vi "Main.vi"() -> ()   [LabVIEW 2021]
doc: "This vi acts as an user interface to display acquire data and save data when required. User can ineract with the panel to choose file (CSV or TDMS) and data display type(chart or graph). It also allow user to select channel index and define channel name, scale and offset. It then can let user choose a moment to start recording either on defined time length or user choice."
uses:
  Control/Data Display Choice Enum.ctl
  Control/File Choice Enum.ctl
  Control/User Interface Reference Cluster.ctl
  Control/Data Display Manager Enum.ctl
  Control/Volt Chl.ctl
  Control/File Manager Enum.ctl
  Control/Command and Data Cluster.ctl
  Control/DAQ Manager Enum.ctl
  <extravilib>/ChannelInstances/Stream-a[.](wfm(dbl))/Read With Abort.vi
  <extravilib>/ChannelInstances/Stream-a[.](wfm(dbl))/Write With Abort.vi
  <extravilib>/ChannelInstances/Stream-a[.](wfm(dbl))/EndpointRead.vi
  <extravilib>/ChannelInstances/Stream-a[.](wfm(dbl))/Endpoint.vi
  <extravilib>/ChannelInstances/Stream-a[.](wfm(dbl))/Instantiate.vi
  <extravilib>/ChannelInstances/Event Messenger-t'Command and Data Cluster.ctl'/Instantiate.vi
  <extravilib>/ChannelInstances/Event Messenger-t'Command and Data Cluster.ctl'/))Channel.vi
  <extravilib>/ChannelInstances/Stream-a[.](wfm(dbl))/)Channel.vi
  <resource>/ChannelSupport/_ChannelSupport/WaitIfNeeded.vi
  <extravilib>/ChannelInstances/Event Messenger-t'Command and Data Cluster.ctl'.lvlib
  <extravilib>/ChannelInstances/Stream-a[.](wfm(dbl)).lvlib
panel:
  out "Error":errorcluster
  out "Overall Raw \nVoltage Mean":dbl[](array[numeric])
  out "Raw Voltage Mean \nper Second":dbl[](array[numeric])
  out "Recording":bool
  in  "File Choice":T1=enum."CSV File"
  in  "DD Choice":T2 caption="Data Display Choice"
  out "File Path":path
  in  "Choice Ok":bool
  in  "File Name":string
  in  "Exit":bool
  in  "Use Re Time":bool caption="Use Record Time"
  in  "Re Time":dbl=10.0 caption="Record Time (s)"
  in  "Device Name":tag
  in  "Sample Rate":i32=100 caption="Sample Rate (S/s)"
  in  "Init Button":bool
  in  "Record":bool
  in  "Start":bool
  in  "Stop":bool
  out "element":waveform(dbl)[](array[waveform])
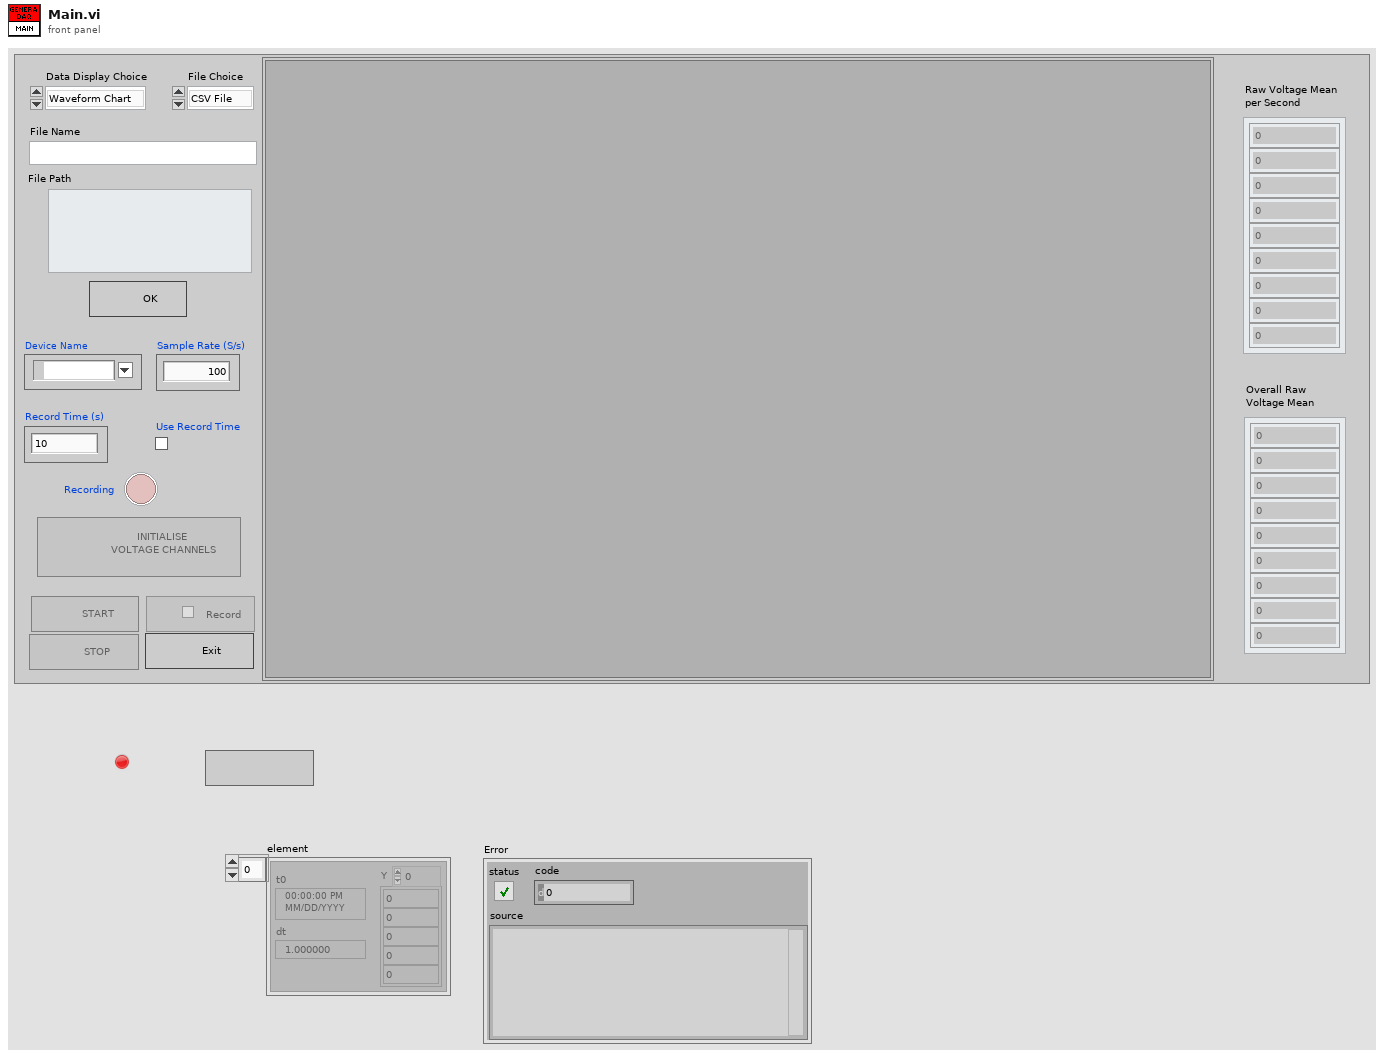
[diagram p1: front panel]
types:
  T1 = typedef "File Choice Enum.ctl" = enum16{"TDMS File", "CSV File"}
  T2 = typedef "Data Display Choice Enum.ctl" = enum16{"Waveform Chart", "Waveform Graph"}
  T3 = typedef "User Interface Reference Cluster.ctl" = cluster{"Choice Ok":refnum<vi>, "Init Button":refnum<vi>, "Start":refnum<vi>, "Record":refnum<vi>, "Stop":refnum<vi>, "Exit":refnum<vi>, "File Choice":refnum<vi>, "DD Choice":refnum<vi>}
  T4 = typedef "Command and Data Cluster.ctl" = cluster{"Command":string, "Data":variant}
  T5 = typedef "Event Messenger-t'Command and Data Cluster.ctl'.lvlib/))Channel.ctl" = refnum<queue>
  T6 = typedef "DAQ Manager Enum.ctl" = enum16{"Config", "Start", "Read", "Stop"}
  T7 = typedef "Volt Chl.ctl" = cluster{"Index":i32[], "Chl Name":string[], "Scale":dbl[], "Offset":dbl[], "Sample Rate":i32, "Device Name":tag, "Channel":tag}
  T8 = typedef "Stream-a[.](wfm(dbl)).lvlib/)Channel.ctl" = refnum<queue>
  T9 = typedef "File Manager Enum.ctl" = enum16{"Create File", "Config Data", "Volt Data", "Set Time", "Close File"}
  T10 = typedef "Data Display Manager Enum.ctl" = enum16{"Display Choice", "Config Data", "Volt Data"}
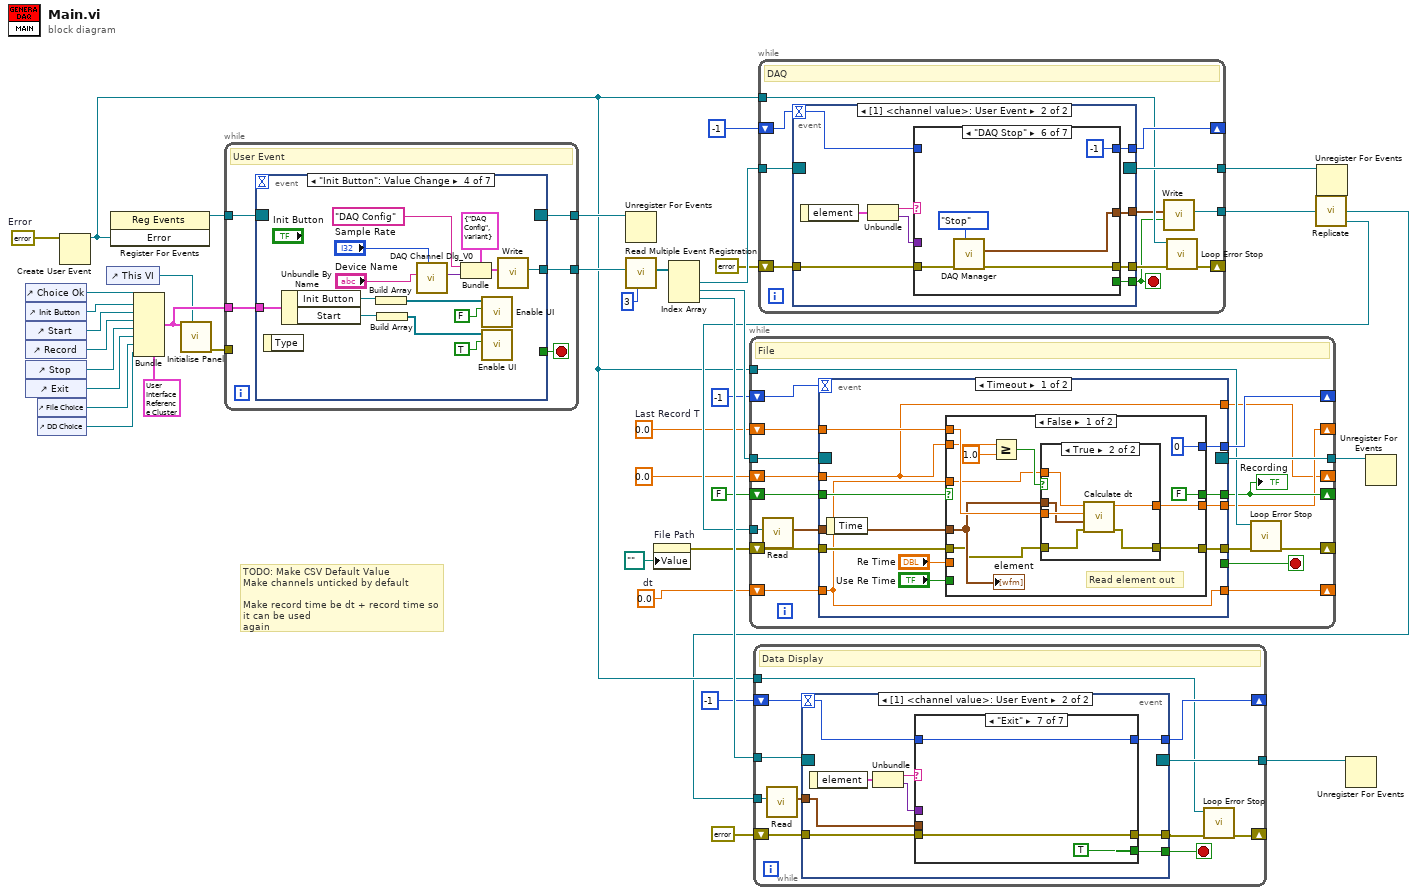
[diagram p0: block diagram]
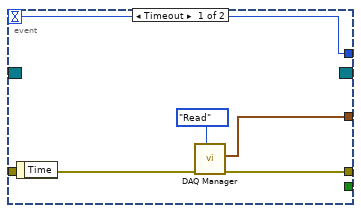
[diagram p2: hidden frame]
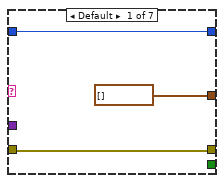
[diagram p3: hidden frame]
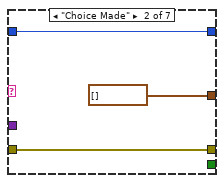
[diagram p4: hidden frame]
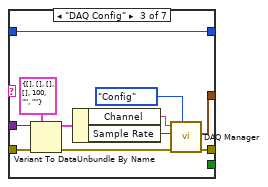
[diagram p5: hidden frame]
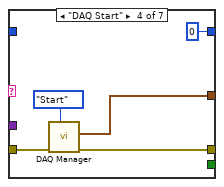
[diagram p6: hidden frame]
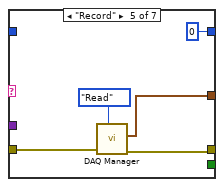
[diagram p7: hidden frame]
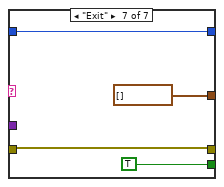
[diagram p8: hidden frame]
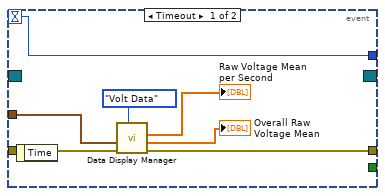
[diagram p9: hidden frame]
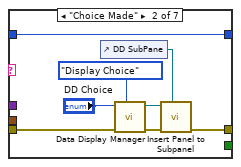
[diagram p11: hidden frame]
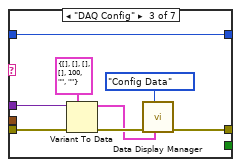
[diagram p12: hidden frame]
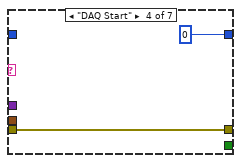
[diagram p13: hidden frame]
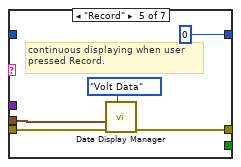
[diagram p14: hidden frame]
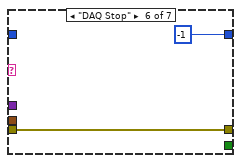
[diagram p15: hidden frame]
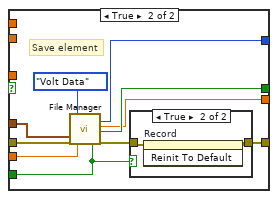
[diagram p17: hidden frame]
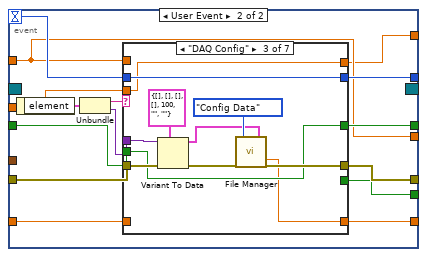
[diagram p19: hidden frame]
diagram:
  w2 = 0.0  # dt
  w3 = 0.0  # Last Record T
  w7 = errorcluster {"status"=FALSE, "code"=0, "source"=""}  # Error
  # "TODO: Make CSV Default Value\nMake channels unticked by default\n\nMake record time be dt + record time so it can be used \nagain"
  n1 = control-ref of="Choice Ok"() -> (w25:refnum<vi>)
  n2 = control-ref of="Init Button"() -> (w24:refnum<vi>)
  n3 = control-ref of="Start"() -> (w23:refnum<vi>)
  n4 = control-ref of="Record"() -> (w22:refnum<vi>)
  n5 = control-ref of="Stop"() -> (w21:refnum<vi>)
  n6 = control-ref of="Exit"() -> (w20:refnum<vi>)
  n7 = control-ref of="File Choice"() -> (w19:refnum<vi>)
  n8 = control-ref of="DD Choice"() -> (w18:refnum<vi>)
  n9 = Create User Event(user event datatype=w7) -> (user event=w10:refnum<user-event>)  [unwired: 1 in, 1 out]
  n10 = control-ref of="This VI"() -> (w8:refnum<vi>)
  n11 = register-events(w10) -> (reference out=w12:refnum<event-registration>)  [unwired: 2 in, 1 out]
  n12 = Bundle(cluster=T3 {"Choice Ok"=refnum, "Init Button"=refnum, "Start"=refnum, "Record"=refnum, "Stop"=refnum, "Exit"=refnum, "File Choice"=refnum, "DD Choice"=refnum} ("output cluster"), "Choice Ok"=w25, "Init Button"=w24, "Start"=w23, "Record"=w22, "Stop"=w21, "Exit"=w20, "File Choice"=w19, "DD Choice"=w18) -> (w15:T3)
  n13 = call "Initialise Panel.vi"("This VI"=w8, "UI Ref"=w15) -> ("error out"=w16:errorcluster)  [unwired: 9 in]
  n14 = while {
    tunnel: [w43] -> w33
    tunnel: w16 -> [_]
    tunnel: w15 -> [w42]
    tunnel: w12 -> [w41]
    tunnel: [w40] -> w11
    stop <- w44 stop-if-true
    # "User Event"
    n15 = event shown="[3] \"Init Button\": Value Change" {
      selector: w41 -> [_ _ _ _ _ _ _]
      dyn-events: [_ _ _ _ _ _ _] -> w40
      timeout: _ -> [_ _ _ _ _ _ _]
      tunnel: [TRUE TRUE _ _ _ _ _] -> w44
      tunnel: [w45 w53 w65 w78 w91 w96 w108] -> w43
      tunnel: w42 -> [_ _ w64 w73 w83 _ w107]
      event "Exit": Value Change {
        n16 = event-data() -> ()  [unwired: 1 in, 1 out]
        n17 = call <extravilib>:"Write.vi"("element"=T4 {"Command"="Exit", "Data"=variant} ("Cluster")) -> ("channel"=w45:T5)  [unwired: 9 in, 1 out]
      }
      event User Event {
        w52 = errorcluster {"status"=FALSE, "code"=0, "source"=""}  # Error
        n18 = event-data() -> ("status"=w51:bool, "code"=w50:i32, "source"=w49:string)  [unwired: 1 in]
        n19 = Bundle(cluster=w52, "status"=w51, "code"=w50, "source"=w49) -> (→"Error":errorcluster)
        n20 = call <extravilib>:"Write.vi"("element"=T4 {"Command"="Exit", "Data"=variant} ("Cluster")) -> ("channel"=w53:T5)  [unwired: 9 in, 1 out]
      }
      event "Choice Ok": Value Change {
        n21 = event-data() -> ()  [unwired: 1 in, 1 out]
        n22 = Unbundle By Name(w64) -> ("File Choice"=w57:refnum<vi>, "DD Choice"=w56:refnum<vi>, "Choice Ok"=w63:refnum<vi>, "Init Button"=w62:refnum<vi>)
        n23 = Build Array(w57, w56, w63) -> (w60:refnum<vi>[])
        n24 = Build Array(w62) -> (w58:refnum<vi>[])
        n25 = call <extravilib>:"Write.vi"("element"=T4 {"Command"="Choice Made", "Data"=variant} ("Cluster")) -> ("channel"=w65:T5)  [unwired: 9 in, 1 out]
        n26 = call "Enable UI.vi"("Enable?"=FALSE, "output cluster"=w60) -> ()  [unwired: 9 in, 1 out]
        n27 = call "Enable UI.vi"("Enable?"=TRUE, "output cluster"=w58) -> ()  [unwired: 9 in, 1 out]
      }
      event "Init Button": Value Change {
        n28 = event-data() -> ()  [unwired: 1 in, 1 out]
        n29 = Unbundle By Name(w73) -> ("Init Button"=w68:refnum<vi>, "Start"=w67:refnum<vi>)
        n30 = Build Array(w68) -> (w72:refnum<vi>[])
        n31 = Build Array(w67) -> (w71:refnum<vi>[])
        n32 = call "DAQ Channel Dlg_V0.vi"("DAQ Sample Rate (S/s)"="Sample Rate", "Device Name"="Device Name") -> ("Chl Infor"=w74:variant)  [unwired: 9 in]
        n33 = Bundle(cluster=T4 {"Command"="DAQ Config", "Data"=variant} ("Cluster"), "Command"="DAQ Config" ("element"), "Data"=w74) -> (w76:T4)
        n34 = call "Enable UI.vi"("Enable?"=FALSE, "output cluster"=w72) -> ()  [unwired: 9 in, 1 out]
        n35 = call "Enable UI.vi"("Enable?"=TRUE, "output cluster"=w71) -> ()  [unwired: 9 in, 1 out]
        n36 = call <extravilib>:"Write.vi"("element"=w76) -> ("channel"=w78:T5)  [unwired: 9 in, 1 out]
      }
      event "Start": Value Change {
        n37 = event-data() -> ()  [unwired: 1 in, 1 out]
        n38 = Unbundle By Name(w83) -> ("Exit"=w81:refnum<vi>, "Start"=w85:refnum<vi>, "Record"=w84:refnum<vi>, "Stop"=w82:refnum<vi>)
        n39 = Build Array(w81, w85) -> (w89:refnum<vi>[])
        n40 = Build Array(w84, w82) -> (w88:refnum<vi>[])
        n41 = call "Enable UI.vi"("Enable?"=FALSE, "output cluster"=w89) -> ()  [unwired: 9 in, 1 out]
        n42 = call "Enable UI.vi"("Enable?"=TRUE, "output cluster"=w88) -> ()  [unwired: 9 in, 1 out]
        n43 = call <extravilib>:"Write.vi"("element"=T4 {"Command"="DAQ Start", "Data"=variant} ("Cluster")) -> ("channel"=w91:T5)  [unwired: 9 in, 1 out]
      }
      event "Record": Value Change {
        n44 = event-data() -> ()  [unwired: 1 in, 1 out]
        n45 = To Variant(anything="Record") -> (Variant=w93:variant)
        n46 = Bundle(cluster=T4 {"Command"="Record", "Data"=variant} ("Cluster"), "Data"=w93) -> (w92:T4)  [unwired: 1 in]
        n47 = call <extravilib>:"Write.vi"("element"=w92) -> ("channel"=w96:T5)  [unwired: 9 in, 1 out]
      }
      event "Stop": Value Change {
        n48 = event-data() -> ()  [unwired: 1 in, 1 out]
        n49 = Unbundle By Name(w107) -> ("Choice Ok"=w103:refnum<vi>, "File Choice"=w104:refnum<vi>, "DD Choice"=w105:refnum<vi>, "Exit"=w101:refnum<vi>, "Record"=w100:refnum<vi>, "Stop"=w97:refnum<vi>)
        n50 = Build Array(w103, w104, w105, w101) -> (w102:refnum<vi>[])
        n51 = Build Array(w100, w97) -> (w98:refnum<vi>[])
        n52 = call "Enable UI.vi"("Enable?"=TRUE, "output cluster"=w102) -> ()  [unwired: 9 in, 1 out]
        n53 = call "Enable UI.vi"("Enable?"=FALSE, "output cluster"=w98) -> ()  [unwired: 9 in, 1 out]
        n54 = call <extravilib>:"Write.vi"("element"=T4 {"Command"="DAQ Stop", "Data"=variant} ("Cluster")) -> ("channel"=w108:T5)  [unwired: 9 in, 1 out]
      }
    }
  }
  n55 = Unregister For Events(event registration refnum=w11) -> ()  [unwired: 1 in, 1 out]
  n56 = call <extravilib>:"Read Multiple Event Registration.vi"("number of event structures"=u16 3, "channel"=w33) -> ("event registration refnums"=w31:refnum<event-registration>[])  [unwired: 9 in]
  n57 = property on="File Path" class="Path"("Value"=path "" ("File Path")) -> (error out=w13:errorcluster)  [unwired: 2 in, 1 out]
  n58 = Index Array(array=w31) -> (element #1=w37:refnum<event-registration>, element #2=w38:refnum<event-registration>, element #3=w36:refnum<event-registration>)  [unwired: 3 in]
  n59 = while {
    tunnel: w37 -> [w120]
    tunnel: [w119] -> w34
    shift-right: [w117] -> _
    shift-left: -1 -> [w118]
    tunnel: [w112] -> w28
    shift-right: [w114] -> _
    shift-left: errorcluster {"status"=FALSE, "code"=0, "source"=""} ("error constant") -> [w116]
    tunnel: w10 -> [w115]
    stop <- w110 stop-if-true
    # "DAQ"
    n60 = event shown="[1] <channel value>: User Event" {
      selector: w120 -> [_ _]
      dyn-events: [_ _] -> w119
      timeout: w118 -> [w125 w129]
      tunnel: [w124 w134] -> w113
      tunnel: [_ w133] -> w110
      tunnel: [w125 w128] -> w117
      tunnel: w116 -> [w122 w127]
      tunnel: [w121 w126] -> w111
      event Timeout {
        n61 = event-data() -> ()  [unwired: 1 in, 1 out]
        n62 = call "DAQ Manager.vi"("Enum"=DAQ_Manager_Enum."Read", "error in"=w122) -> ("error out"=w124:errorcluster, "data"=w121:waveform(dbl)[])  [unwired: 8 in]
      }
      event User Event {
        n63 = event-data() -> ("element"=w132:T4)  [unwired: 1 in]
        n64 = Unbundle(w132) -> ("Command"=w131:string, "Data"=w130:variant)
        n65 = case shown="\"DAQ Stop\"" w131 {
          tunnel: [w136 w139 w144 w155 w157 w164 w168] -> w134
          tunnel: [_ _ _ _ _ _ TRUE] -> w133
          tunnel: w130 -> [_ _ w151 _ _ _ _]
          tunnel: w129 -> [w137 w140 w143 _ _ _ w170]
          tunnel: [w137 w140 w143 0 0 -1 w170] -> w128
          tunnel: w127 -> [w136 w139 w142 w153 w158 w163 w168]
          tunnel: [waveform(dbl)[] [] ("element") waveform(dbl)[] [] ("element") w141 w152 w159 w162 waveform(dbl)[] [] ("element")] -> w126
          frame Default {
          }
          frame "Choice Made" {
          }
          frame "DAQ Config" {
            n66 = Variant To Data(error in=w142, type=T7 {"Index"=[], "Chl Name"=[], "Scale"=[], "Offset"=[], "Sample Rate"=100, "Device Name"="", "Channel"=""} ("Volt Channel"), Variant=w151) -> (data=w149:T7, error out=w146:errorcluster)
            n67 = Unbundle By Name(w149) -> ("Channel"=w148:tag, "Sample Rate"=w147:i32)
            n68 = call "DAQ Manager.vi"("Enum"=DAQ_Manager_Enum."Config", "error in"=w146, "Sample Rate"=w147, "Chl"=w148) -> ("error out"=w144:errorcluster, "data"=w141:waveform(dbl)[])  [unwired: 6 in]
          }
          frame "DAQ Start" {
            n69 = call "DAQ Manager.vi"("Enum"=DAQ_Manager_Enum."Start", "error in"=w153) -> ("error out"=w155:errorcluster, "data"=w152:waveform(dbl)[])  [unwired: 8 in]
          }
          frame "Record" {
            n70 = call "DAQ Manager.vi"("Enum"=DAQ_Manager_Enum."Read", "error in"=w158) -> ("error out"=w157:errorcluster, "data"=w159:waveform(dbl)[])  [unwired: 8 in]
          }
          frame "DAQ Stop" {
            n71 = call "DAQ Manager.vi"("Enum"=DAQ_Manager_Enum."Stop", "error in"=w163) -> ("error out"=w164:errorcluster, "data"=w162:waveform(dbl)[])  [unwired: 8 in]
          }
          frame "Exit" {
          }
        }
      }
    }
    n72 = call <extravilib>:"Write.vi"("last element? (F)"=w110, "element"=w111) -> ("channel"=w112:T8)  [unwired: 7 in, 2 out]
    n73 = call "Loop Error Stop.vi"("error in"=w113, "user event"=w115) -> ("error out"=w114:errorcluster)  [unwired: 9 in]
  }
  n74 = call <extravilib>:"Replicate.vi"("stream"=w28) -> ("stream copy 1"=w9:T8, "stream copy 2"=w27:T8)  [unwired: 7 in]
  n75 = while {
    tunnel: w38 -> [w189]
    tunnel: [w188] -> w39
    tunnel: w27 -> [w186]
    shift-right: [w179] -> _
    shift-left: w13 -> [w185]
    shift-right: [w182] -> _
    shift-left: -1 -> [w183]
    shift-right: [w177] -> _
    shift-left: FALSE ("Recording") -> [w181]
    tunnel: w10 -> [w178]
    shift-right: [w175] -> _
    shift-left: w3 -> [w176]
    shift-right: [w173] -> _
    shift-left: w2 -> [w174]
    shift-right: [w171] -> _
    shift-left: 0.0 -> [w172]
    stop <- w187 stop-if-true
    # "File"
    n76 = call <extravilib>:"Read.vi"("channel"=w186) -> ("element"=w184:waveform(dbl)[])  [unwired: 6 in, 4 out]
    n77 = event shown="[0] Timeout" {
      selector: w189 -> [_ _]
      dyn-events: [_ _] -> w188
      timeout: w183 -> [_ w242]
      tunnel: [w200 w248] -> w180
      tunnel: [_ w247] -> w187
      tunnel: w185 -> [w201 w243]
      tunnel: w184 -> [w199 _]
      tunnel: [w196 w241] -> w182
      tunnel: [w194 w240] -> w177
      tunnel: w181 -> [w198 w239]
      tunnel: w176 -> [w192 w238]
      tunnel: [w193 w238] -> w175
      tunnel: w174 -> [w190 w236]
      tunnel: [w190 w237] -> w173
      tunnel: w172 -> [w191 w234]
      tunnel: [w191 w235] -> w171
      event Timeout {
        n78 = event-data() -> ()  [unwired: 1 in, 1 out]
        n79 = case shown="False" w198 {
          tunnel: w201 -> [w207 w230]
          tunnel: [w206 w223] -> w200
          tunnel: w199 -> [w208 w228]
          tunnel: "Re Time" -> [_ w227]
          tunnel: [0 ("timeout") w226] -> w196
          tunnel: "Use Re Time" -> [_ w222]
          tunnel: [FALSE ("Recording") w225] -> w194
          tunnel: [w209 w221] -> w193
          tunnel: w192 -> [w210 _]
          tunnel: w191 -> [w205 _]
          tunnel: w190 -> [w202 _]
          frame False {
            # "Read element out"
            n80 = Greater Or Equal?(x=w205, y=1.0) -> (x >= y?=w203:bool)
            n81 = case shown="True" w203 {
              tunnel: w210 -> [w214 w220]
              tunnel: [w214 w219] -> w209
              tunnel: w208 -> [_ w218]
              tunnel: w207 -> [w213 w217]
              tunnel: [w213 w216] -> w206
              tunnel: w202 -> [_ w215]
              frame False {
              }
              frame True {
                n82 = call "Calculate dt.vi"("error in"=w217, "Voltage in"=w218, "t_start in"=w220, "dt"=w215) -> ("error out"=w216:errorcluster, "t_start out"=w219:dbl)  [unwired: 6 in]
              }
            }
            "element" <- w208
          }
          frame True {
            # "Save element"
            n83 = call "File Manager.vi"("Voltage"=w228, "error in"=w230, "Enum"=File_Manager_Enum."Volt Data", "Record Time (s)"=w227, "Use Record Time"=w222) -> ("timeout"=w226:i32, "ET out"=w221:dbl, "Recording"=w225:bool, "error out"=w224:errorcluster)  [unwired: 9 in, 2 out]
            n84 = case shown="True" w222 {
              tunnel: w224 -> [w231 w233]
              tunnel: [w231 w232] -> w223
              frame False {
              }
              frame True {
                n85 = invoke on="Record" class="Bool (strict)" method="Reinit To Default"(error in=w233) -> (error out=w232:errorcluster)  [unwired: 2 in, 2 out]
              }
            }
          }
        }
      }
      event User Event {
        n86 = event-data() -> ("element"=w246:T4)  [unwired: 1 in]
        n87 = Unbundle(w246) -> ("Command"=w245:string, "Data"=w244:variant)
        n88 = case shown="\"DAQ Config\"" w245 {
          tunnel: [w252 w261 w273 w279 w283 w293 w301] -> w248
          tunnel: [_ _ _ _ _ _ TRUE] -> w247
          tunnel: w244 -> [_ _ w272 _ w289 _ _]
          tunnel: w243 -> [w252 w257 w268 w279 w288 w294 w301]
          tunnel: w242 -> [w253 w258 w267 _ _ _ w303]
          tunnel: [w253 w258 w267 0 0 -1 w303] -> w241
          tunnel: [w251 w256 w266 w277 w287 FALSE w300] -> w240
          tunnel: w239 -> [w251 w256 w266 w277 _ _ w300]
          tunnel: w238 -> [_ _ _ _ w282 _ _]
          tunnel: [w250 w255 w265 w276 w281 w292 w299] -> w237
          tunnel: w236 -> [w250 w255 _ w276 w281 w292 w299]
          tunnel: [w249 w254 w264 w275 1.0 w291 w298] -> w235
          tunnel: w234 -> [w249 w254 w264 w275 _ w291 w298]
          frame Default {
          }
          frame "Choice Made" {
            n89 = call "File Manager.vi"("File Name"="File Name", "File Choice"="File Choice", "error in"=w257, "Enum"=File_Manager_Enum."Create File") -> ("File Path"=→"File Path":path, "error out"=w261:errorcluster)  [unwired: 10 in, 4 out]
          }
          frame "DAQ Config" {
            n90 = Variant To Data(error in=w268, type=T7 {"Index"=[], "Chl Name"=[], "Scale"=[], "Offset"=[], "Sample Rate"=100, "Device Name"="", "Channel"=""} ("Volt Channel"), Variant=w272) -> (data=w269:T7, error out=w270:errorcluster)
            n91 = call "File Manager.vi"("error in"=w270, "Enum"=File_Manager_Enum."Config Data", "Volt Channel"=w269) -> ("dt Out"=w265:dbl, "error out"=w273:errorcluster)  [unwired: 11 in, 4 out]
          }
          frame "DAQ Start" {
          }
          frame "Record" {
            # "output 1 to n"
            n92 = Variant To Data(error in=w288, type=TRUE, Variant=w289) -> (data=w287:bool, error out=w284:errorcluster)
            n93 = call "File Manager.vi"("Existing Time"=w282, "error in"=w284, "Enum"=File_Manager_Enum."Set Time") -> ("error out"=w283:errorcluster)  [unwired: 11 in, 5 out]
          }
          frame "DAQ Stop" {
            n94 = call "File Manager.vi"("error in"=w294, "Enum"=File_Manager_Enum."Close File") -> ("error out"=w293:errorcluster)  [unwired: 12 in, 5 out]
          }
          frame "Exit" {
          }
        }
      }
    }
    "Recording" <- w177
    n95 = call "Loop Error Stop.vi"("error in"=w180, "user event"=w178) -> ("error out"=w179:errorcluster)  [unwired: 9 in]
  }
  n96 = while {
    tunnel: w36 -> [w314]
    tunnel: [w313] -> w35
    shift-right: [w310] -> _
    shift-left: -1 -> [w311]
    tunnel: w9 -> [w309]
    shift-right: [w305] -> _
    shift-left: errorcluster {"status"=FALSE, "code"=0, "source"=""} ("error constant") -> [w307]
    tunnel: w10 -> [w304]
    stop <- w312 stop-if-true
    # "Data Display"
    n97 = call <extravilib>:"Read.vi"("channel"=w309) -> ("element"=w308:waveform(dbl)[])  [unwired: 6 in, 4 out]
    n98 = event shown="[1] <channel value>: User Event" {
      selector: w314 -> [_ _]
      dyn-events: [_ _] -> w313
      timeout: w311 -> [w317 w325]
      tunnel: [_ w330] -> w312
      tunnel: [w321 w329] -> w306
      tunnel: [w317 w324] -> w310
      tunnel: w308 -> [w319 w322]
      tunnel: w307 -> [w318 w323]
      event Timeout {
        n99 = event-data() -> ()  [unwired: 1 in, 1 out]
        n100 = call "Data Display Manager.vi"("Enum"=Data_Display_Manager_Enum."Volt Data", "error in"=w318, "Raw Data"=w319) -> ("error out"=w321:errorcluster, "Overall Mean"=→"Overall Raw \nVoltage Mean":dbl[], "Mean per Second"=→"Raw Voltage Mean \nper Second":dbl[])  [unwired: 5 in, 1 out]
      }
      event User Event {
        n101 = event-data() -> ("element"=w328:T4)  [unwired: 1 in]
        n102 = Unbundle(w328) -> ("Command"=w327:string, "Data"=w326:variant)
        n103 = case shown="\"Exit\"" w327 {
          tunnel: [_ _ _ _ _ _ TRUE] -> w330
          tunnel: [w331 w335 w346 w349 w351 w356 w358] -> w329
          tunnel: w326 -> [_ _ w344 _ _ _ _]
          tunnel: w325 -> [w332 w334 w348 _ _ _ w359]
          tunnel: [w332 w334 w348 0 0 -1 w359] -> w324
          tunnel: w323 -> [w331 w333 w341 w349 w352 w356 w358]
          tunnel: w322 -> [_ _ _ _ w353 _ _]
          frame Default {
          }
          frame "Choice Made" {
            n104 = control-ref of="DD SubPane"() -> (w338:refnum<vi>)
            n105 = call "Data Display Manager.vi"("Enum"=Data_Display_Manager_Enum."Display Choice", "error in"=w333, "Data Display Choice"="DD Choice") -> ("error out"=w336:errorcluster, "VI Ref"=w337:refnum<vi>)  [unwired: 5 in, 2 out]
            n106 = call "Insert Panel to Subpanel.vi"("SubPanel in"=w338, "error in"=w336, "VI Ref"=w337) -> ("error out"=w335:errorcluster)  [unwired: 8 in]
          }
          frame "DAQ Config" {
            n107 = Variant To Data(error in=w341, type=T7 {"Index"=[], "Chl Name"=[], "Scale"=[], "Offset"=[], "Sample Rate"=100, "Device Name"="", "Channel"=""} ("Volt Channel"), Variant=w344) -> (data=w342:T7, error out=w343:errorcluster)
            n108 = call "Data Display Manager.vi"("Volt Channel"=w342, "Enum"=Data_Display_Manager_Enum."Config Data", "error in"=w343) -> ("error out"=w346:errorcluster)  [unwired: 5 in, 3 out]
          }
          frame "DAQ Start" {
          }
          frame "Record" {
            # "continuous displaying when user\npressed Record."
            n109 = call "Data Display Manager.vi"("Enum"=Data_Display_Manager_Enum."Volt Data", "error in"=w352, "Raw Data"=w353) -> ("error out"=w351:errorcluster)  [unwired: 5 in, 3 out]
          }
          frame "DAQ Stop" {
          }
          frame "Exit" {
          }
        }
      }
    }
    n110 = call "Loop Error Stop.vi"("error in"=w306, "user event"=w304) -> ("error out"=w305:errorcluster)  [unwired: 9 in]
  }
  n111 = Unregister For Events(event registration refnum=w34) -> ()  [unwired: 1 in, 1 out]
  n112 = Unregister For Events(event registration refnum=w35) -> ()  [unwired: 1 in, 1 out]
  n113 = Unregister For Events(event registration refnum=w39) -> ()  [unwired: 1 in, 1 out]
